vi "Read BaseNode ID.vi"(8 "error in (no error)":errorcluster, 11 "Scalar Bitpacking Testing in":refnum<class "FPGA Addon Scalar Bitpacking Unit Tests.lvclass">=refnum) -> (0 "error out":errorcluster, 2 "BaseNode ID":u64, 3 "Scalar Bitpacking Testing out":refnum<class "FPGA Addon Scalar Bitpacking Unit Tests.lvclass">)   [LabVIEW 2019, in "FPGA Addon Scalar Bitpacking Unit Tests.lvclass"]
uses:
  FPGA Addon Scalar Bitpacking Unit Tests.lvclass
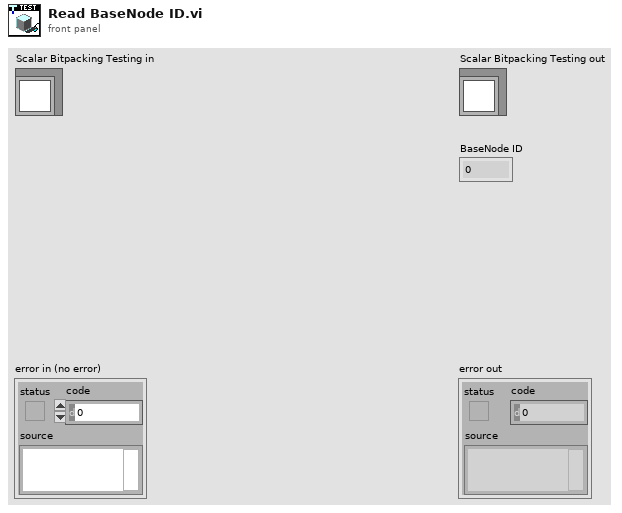
[diagram p1: front panel]
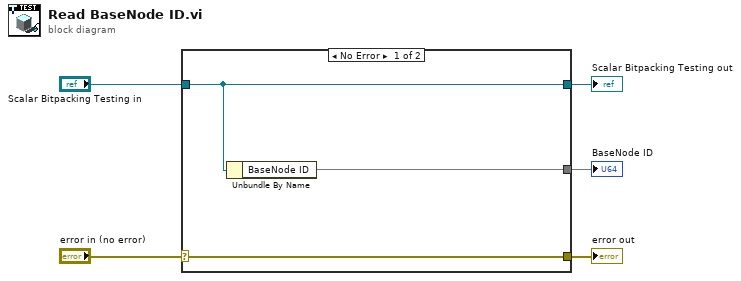
[diagram p0: block diagram]
diagram:
  n1 = case shown="No Error" "error in (no error)" {
    selector: "error in (no error)" -> [w8 w9]
    tunnel: [w8 w9] -> w4
    tunnel: [w7 w10] -> w2
    tunnel: "Scalar Bitpacking Testing in" -> [w7 w10]
    tunnel: [w6 _] -> w1
    frame No Error {
      n2 = Unbundle By Name(w7) -> ("BaseNode ID"=w6)
    }
    frame Error {
    }
  }
  "error out" <- w4
  "Scalar Bitpacking Testing out" <- w2
  "BaseNode ID" <- w1
